vi "Degrisse commande image si sourie relache.vi"(8 "error in (no error)":errorcluster caption="entrée d'erreur (pas d'erreur)", 10 "Nom commande":string[](array[string]), 11 "VI en entrée":refnum<vi>) -> (0 "error out":errorcluster caption="sortie d'erreur")   [LabVIEW 2020]
panel:
  in  "Commande onglets":enum32{"Page 1", "Page 2"}(tab)
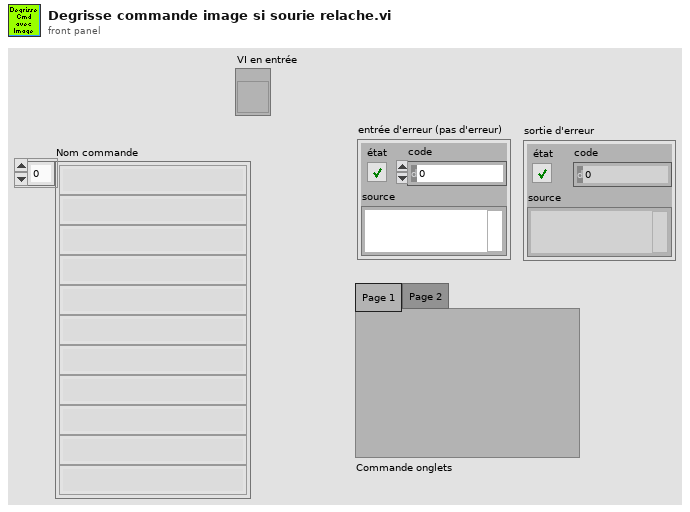
[diagram p1: front panel]
types:
  T1 = enum8{"Enabled", "Disabled", "Disabled and Grayed Out"}
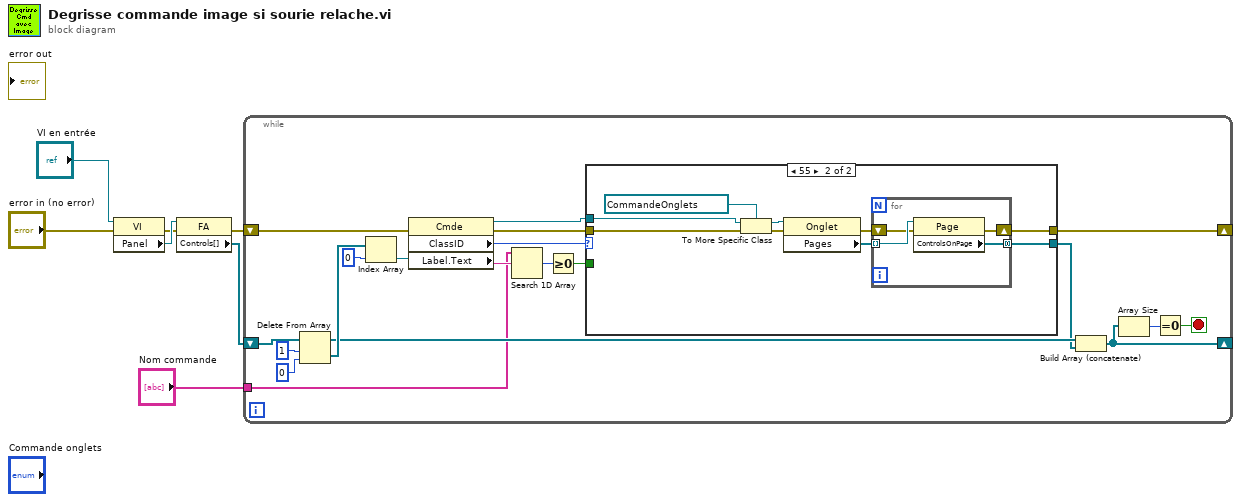
[diagram p0: block diagram]
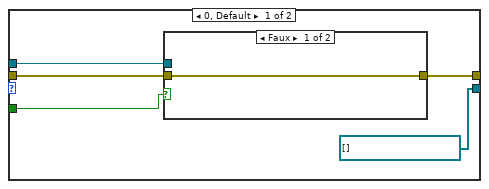
[diagram p2: hidden frame]
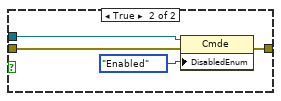
[diagram p3: hidden frame]
diagram:
  n1 = property class="VI"(reference="VI en entrée", error in="error in (no error)") -> (error out=w3:errorcluster, "Panel"=w6:refnum<vi>)  [unwired: 1 out]
  n2 = property class="FA"(reference=w6, error in=w3) -> (error out=w2:errorcluster, "Controls[]"=w7:refnum<vi>[])  [unwired: 1 out]
  n3 = while {
    shift-right: [w11] -> _
    shift-left: w7 -> [w24]
    shift-right: [w16] -> _
    shift-left: w2 -> [w17]
    tunnel: "Nom commande" -> [w14]
    stop <- w10 stop-if-true
    n4 = Delete From Array(array=w24, length=1 ("longueur"), index=0 ("indice")) -> (deleted portion=w21:refnum<vi>[], array with subset deleted=w18:refnum<vi>[])
    n5 = Index Array(array=w21, index=0 ("indice")) -> (element=w19:refnum<vi>)
    n6 = property class="Cmde"(reference=w19, error in=w17) -> (reference out=w27:refnum<vi>, error out=w26:errorcluster, "ClassID"=w25:u32, "Label.Text"=w15:string)
    n7 = Search 1D Array(1D array=w14, element=w15) -> (index of element=w13:i32)  [unwired: 1 in]
    n8 = Greater Or Equal To 0?(x=w13) -> (x >= 0?=w8:bool)
    n9 = case shown="55" w25 {
      tunnel: w27 -> [w32 w45]
      tunnel: w26 -> [w31 w44]
      tunnel: [refnum<vi>[] [] ("ControlsOnPage") w39] -> w9
      tunnel: [w29 w38] -> w16
      tunnel: w8 -> [w28 _]
      frame 0, Default {
        n10 = case shown="Faux" w28 {
          tunnel: w32 -> [_ w37]
          tunnel: w31 -> [w33 w36]
          tunnel: [w33 w34] -> w29
          frame False {
          }
          frame True {
            n11 = property class="Cmde"(reference=w37, error in=w36, "DisabledEnum"=T1."Enabled" ("Désactivé")) -> (error out=w34:errorcluster)  [unwired: 1 out]
          }
        }
      }
      frame 55 {
        n12 = To More Specific Class(target class=refnum<vi> refnum ("Commande onglets"), reference=w45, error in=w44) -> (specific class reference=w43:refnum<vi>, error out=w42:errorcluster)
        n13 = property class="Onglet"(reference=w43, error in=w42) -> (error out=w40:errorcluster, "Pages"=w41:refnum<vi>[])  [unwired: 1 out]
        n14 = for {
          tunnel: w41 -> [w50] mode=indexing
          shift-right: [w48] -> w38
          shift-left: w40 -> [w49]
          tunnel: [w47] -> w39 mode=concatenating
          n15 = property class="Page"(reference=w50, error in=w49) -> (error out=w48:errorcluster, "ControlsOnPage"=w47:refnum<vi>[])  [unwired: 1 out]
        }
      }
    }
    n16 = Build Array (concatenate)(w18, w9) -> (w11:refnum<vi>[])
    n17 = Array Size(array=w11) -> (size(s)=w12:i32)
    n18 = Equal To 0?(x=w12) -> (x = 0?=w10:bool)
  }
